vi "Master.vi"() -> ()   [LabVIEW 2014]
panel:
  in  "정지":bool
  out "Waveform Graph":dbl[](graph)
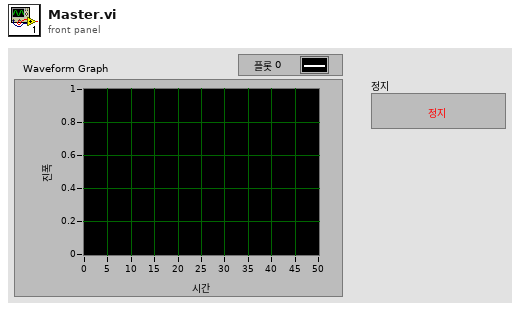
[diagram p1: front panel]
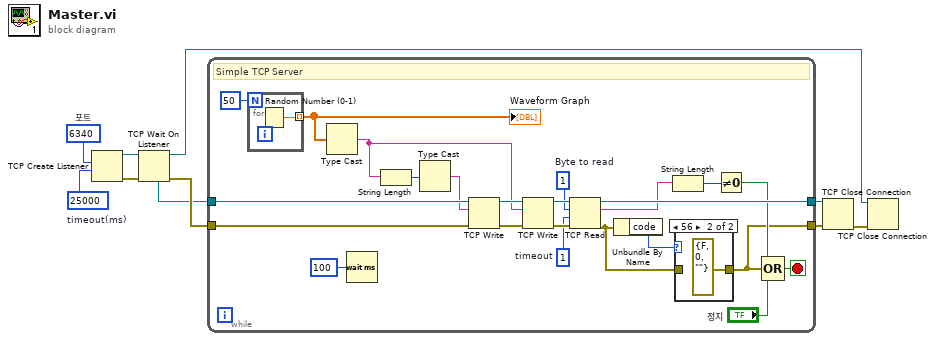
[diagram p0: block diagram]
diagram:
  w7 = 25000  # timeout(ms)
  w8 = u16 6340  # 포트
  n1 = TCP Create Listener(9:w7, 10:w8) -> (0:w10:errorcluster, 3:w9:refnum<k5>)  [unwired: 3 in, 1 out]
  n2 = TCP Wait On Listener(8:w10, 11:w9) -> (0:w6:errorcluster, 3:w1:refnum<k5>, 4:w3:refnum<k5>)  [unwired: 2 in, 2 out]
  n3 = while {
    tunnel: w6 -> [w31]
    tunnel: w3 -> [w33]
    tunnel: [w24] -> w5
    tunnel: [w13] -> w4
    stop <- w17 stop-if-true
    w20 = 1  # timeout
    w21 = 1  # Byte to read
    # "Simple TCP Server"
    n4 = for {
      N: 50 -> [_]
      tunnel: [w36] -> w29 mode=indexing
      n5 = Random Number (0-1)() -> (number: 0 to 1=w36:dbl)
    }
    "Waveform Graph" <- w29
    n6 = Type Cast(x=w29) -> (*(type *) &x=w22:string)  [unwired: 1 in]
    n7 = Wait (ms)(milliseconds to wait=u32 100 ("대기 시간(ms)")) -> ()  [unwired: 1 out]
    n8 = String Length(string=w22) -> (length=w28:i32)
    n9 = Type Cast(x=w28) -> (*(type *) &x=w23:string)  [unwired: 1 in]
    n10 = TCP Write(connection ID=w33, data in=w23, error in (no error)=w31) -> (connection ID out=w32:refnum<k5>, error out=w27:errorcluster)  [unwired: 1 in, 1 out]
    n11 = TCP Write(connection ID=w32, data in=w22, error in (no error)=w27) -> (connection ID out=w25:refnum<k5>, error out=w26:errorcluster)  [unwired: 1 in, 1 out]
    n12 = TCP Read(connection ID=w25, bytes to read=w21, error in (no error)=w26, 9:w20) -> (connection ID out=w24:refnum<k5>, data out=w19:string, error out=w14:errorcluster)  [unwired: 1 in]
    n13 = Unbundle By Name(w14) -> ("code"=w15:i32)
    n14 = String Length(string=w19) -> (length=w18:i32)
    n15 = case shown="56" w15 {
      tunnel: w14 -> [w34 _]
      tunnel: [w34 errorcluster {"status"=FALSE, "code"=0, "source"=""} ("에러 상수")] -> w13
      frame Default {
      }
      frame 56 {
      }
    }
    n16 = Not Equal To 0?(x=w18) -> (x != 0?=w16:bool)
    n17 = Compound Arithmetic op=OR(w16, w13, "정지") -> (w17:bool)
  }
  n18 = TCP Close Connection(connection ID=w5, error in (no error)=w4) -> (error out=w2:errorcluster)  [unwired: 1 in, 1 out]
  n19 = TCP Close Connection(connection ID=w1, error in (no error)=w2) -> ()  [unwired: 1 in, 2 out]
